vi "Numeric Display Format.vi"() -> ()   [LabVIEW 2020]
panel:
  out "Custom (Advanced)":i32=17 format="There are %d apples on the tree."
  in  "Input (I32)":i32=17
  out "Binary":i32=17 format="%b"
  out "Octal":i32=17 format="%o"
  out "Hexadecimal":i32=17 format="%x"
  out "Decimal":i32=17
  out "SI Notation":dbl=10000009.0 format="%#_6p"
  out "Scientific":dbl=10000009.0 format="%#_6e"
  out "Automatic":dbl=10000009.0
  out "Floating Point":dbl=10000009.0
  in  "Number Input (DBL)":dbl=10000009.0
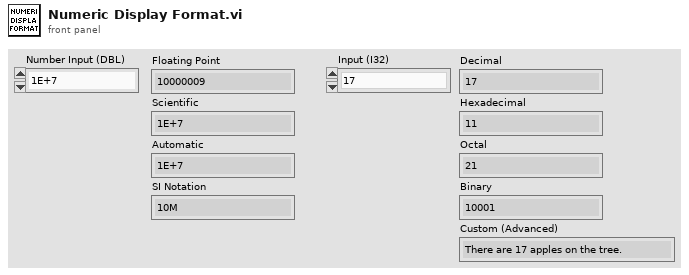
[diagram p1: front panel]
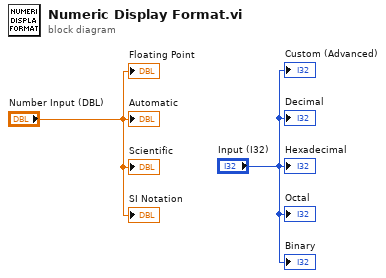
[diagram p0: block diagram]
diagram:
  "Floating Point" <- "Number Input (DBL)"
  "Automatic" <- "Number Input (DBL)"
  "Scientific" <- "Number Input (DBL)"
  "SI Notation" <- "Number Input (DBL)"
  "Decimal" <- "Input (I32)"
  "Hexadecimal" <- "Input (I32)"
  "Octal" <- "Input (I32)"
  "Binary" <- "Input (I32)"
  "Custom (Advanced)" <- "Input (I32)"
